vi "ROI info.vi"(6 "ROI info in":T7={"beads track"=[], "Public"={"标题名"="", "文件路径"=path "", "通道名"=[], "ROI Descriptor out"={"Global Rectangle"=[], "Contours"=[]}, "cali end"=0.0, "array piezo"=[], "LUT_R"=[], " ROI descriptors "=[{"Global Rectangle"=[0, 0, 0, 0], "Contours"=[{"ID"=enum."External", "Type"=12, "Coordinates"=[0, 0, 0, 0, 0]}]}, {"Global Rectangle"=[26, 104, 126, 204], "Contours"=[{"ID"=enum."External", "Type"=12, "Coordinates"=[26, 104, 126, 204, 0]}]}, {"Global Rectangle"=[99, 99, 201, 201], "Contours"=[{"ID"=enum."External", "Type"=12, "Coordinates"=[200, 200, 100, 100, 0]}]}], "tdms ref"=refnum, "分子长度(um)"=0.0, "ROI num"=0, "ROI size num"=[], "测量模式"=enum."force clamp"}, "beads info"=[]} {"Public"."ROI descriptors"."Contours"."Type" items=["No Selection", "Point", "Line", "Rectangle", "Oval", "Polygon", "Freehand Region", "Annulus", "Unused2", "Unused3", "Broken Line", "Freehand Line", "Rotated Rectangle"]; "Public"."ROI Descriptor out"."Contours"."Type" items=["No Selection", "Point", "Line", "Rectangle", "Oval", "Polygon", "Freehand Region", "Annulus", "Unused2", "Unused3", "Broken Line", "Freehand Line", "Rotated Rectangle"]; "beads track"."centroid"."Y Centroid" format="%.2f"; "beads track"."centroid"."X Centroid" format="%.2f"; "beads track"."ROI Des out"."Contours"."Type" items=["No Selection", "Point", "Line", "Rectangle", "Oval", "Polygon", "Freehand Region", "Annulus", "Unused2", "Unused3", "Broken Line", "Freehand Line", "Rotated Rectangle"]}, 7 "action":T8, 8 "error in (no error)":errorcluster caption="错误输入（无错误）", 9 "Public":T1={"标题名"="", "文件路径"=path "", "通道名"=[], "ROI Descriptor out"={"Global Rectangle"=[], "Contours"=[]}, "cali end"=0.0, "array piezo"=[], "LUT_R"=[], " ROI descriptors "=[{"Global Rectangle"=[0, 0, 0, 0], "Contours"=[{"ID"=enum."External", "Type"=12, "Coordinates"=[0, 0, 0, 0, 0]}]}, {"Global Rectangle"=[26, 104, 126, 204], "Contours"=[{"ID"=enum."External", "Type"=12, "Coordinates"=[26, 104, 126, 204, 0]}]}, {"Global Rectangle"=[99, 99, 201, 201], "Contours"=[{"ID"=enum."External", "Type"=12, "Coordinates"=[200, 200, 100, 100, 0]}]}], "tdms ref"=refnum, "分子长度(um)"=0.0, "ROI num"=0, "ROI size num"=[], "测量模式"=enum."force clamp"} {"ROI descriptors"."Contours"."Type" items=["No Selection", "Point", "Line", "Rectangle", "Oval", "Polygon", "Freehand Region", "Annulus", "Unused2", "Unused3", "Broken Line", "Freehand Line", "Rotated Rectangle"]; "ROI Descriptor out"."Contours"."Type" items=["No Selection", "Point", "Line", "Rectangle", "Oval", "Polygon", "Freehand Region", "Annulus", "Unused2", "Unused3", "Broken Line", "Freehand Line", "Rotated Rectangle"]}, 10 "beads track":T6[](array[typedef]) {"centroid"."Y Centroid" format="%.2f"; "centroid"."X Centroid" format="%.2f"; "ROI Des out"."Contours"."Type" items=["No Selection", "Point", "Line", "Rectangle", "Oval", "Polygon", "Freehand Region", "Annulus", "Unused2", "Unused3", "Broken Line", "Freehand Line", "Rotated Rectangle"]}, 11 "beads info":T4[](array[typedef])) -> (0 "error out":errorcluster caption="错误输出", 2 "ROI info out":T7={"beads track"=[], "Public"={"标题名"="", "文件路径"=path "", "通道名"=[], "ROI Descriptor out"={"Global Rectangle"=[], "Contours"=[]}, "cali end"=0.0, "array piezo"=[], "LUT_R"=[], " ROI descriptors "=[{"Global Rectangle"=[0, 0, 0, 0], "Contours"=[{"ID"=enum."External", "Type"=12, "Coordinates"=[0, 0, 0, 0, 0]}]}, {"Global Rectangle"=[26, 104, 126, 204], "Contours"=[{"ID"=enum."External", "Type"=12, "Coordinates"=[26, 104, 126, 204, 0]}]}, {"Global Rectangle"=[99, 99, 201, 201], "Contours"=[{"ID"=enum."External", "Type"=12, "Coordinates"=[200, 200, 100, 100, 0]}]}], "tdms ref"=refnum, "分子长度(um)"=0.0, "ROI num"=0, "ROI size num"=[], "测量模式"=enum."force clamp"}, "beads info"=[]} {"Public"."ROI descriptors"."Contours"."Type" items=["No Selection", "Point", "Line", "Rectangle", "Oval", "Polygon", "Freehand Region", "Annulus", "Unused2", "Unused3", "Broken Line", "Freehand Line", "Rotated Rectangle"]; "Public"."ROI Descriptor out"."Contours"."Type" items=["No Selection", "Point", "Line", "Rectangle", "Oval", "Polygon", "Freehand Region", "Annulus", "Unused2", "Unused3", "Broken Line", "Freehand Line", "Rotated Rectangle"]; "beads track"."centroid"."Y Centroid" format="%.2f"; "beads track"."centroid"."X Centroid" format="%.2f"; "beads track"."ROI Des out"."Contours"."Type" items=["No Selection", "Point", "Line", "Rectangle", "Oval", "Polygon", "Freehand Region", "Annulus", "Unused2", "Unused3", "Broken Line", "Freehand Line", "Rotated Rectangle"]})   [LabVIEW 2017]
doc: "本VI 是功能性全局变量，用来代替ROI info 四处乱跑的局域变量。\n暂时有初始化，读，写 3个功能。\nVI必须被设置为不可重入，以免出现执行中篡改的现象。"
uses:
  Bead info action.ctl
  vision test/ROI info.ctl
  Bead track.ctl
  beads public.ctl
  record mode.ctl
  bead info.ctl
  <vilib>/vision/Image Controls.llb/IMAQ Image.ctl
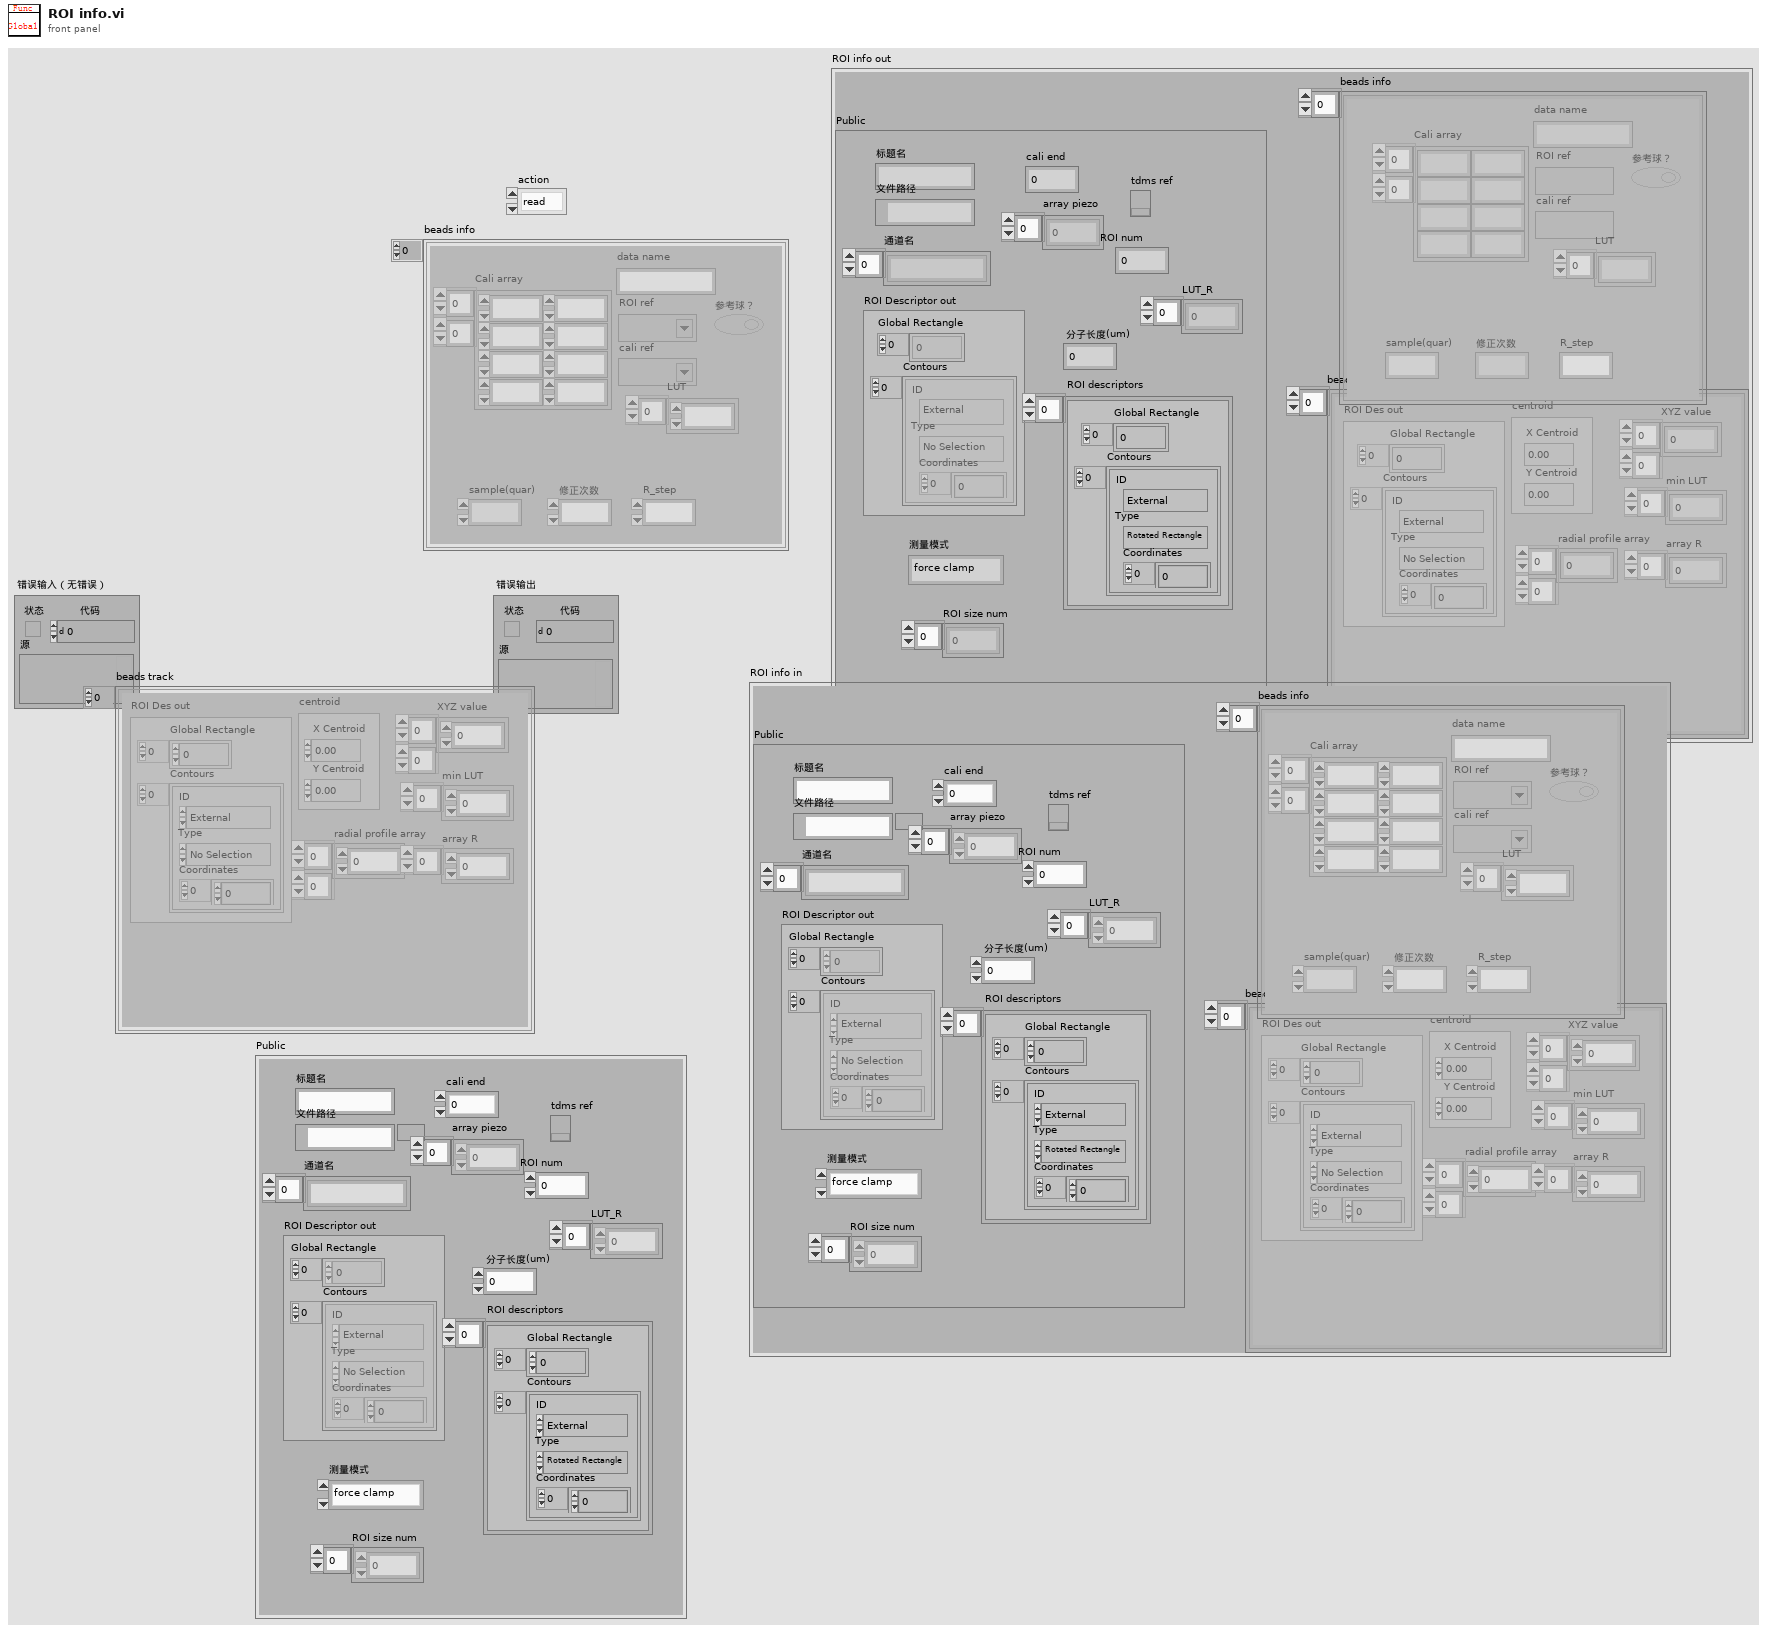
[diagram p1: front panel]
types:
  T1 = typedef "beads public.ctl" = cluster{"标题名":string, "文件路径":path, "通道名":string[], "ROI Descriptor out":T2, "cali end":dbl, "array piezo":dbl[], "LUT_R":dbl[], " ROI descriptors ":T2[], "tdms ref":refnum<k34>, "分子长度(um)":dbl, "ROI num":i32, "ROI size num":i32[], "测量模式":T3}
  T2 = typedef "ROI Descriptor" = cluster{"Global Rectangle":i32[], "Contours":cluster{"ID":enum32{"External", "Internal"}, "Type":u32, "Coordinates":i32[]}[]}
  T3 = typedef "record mode.ctl" = enum16{"force ramp", "force clamp", "user-defined", "force-mixed"}
  T4 = typedef "bead info.ctl" = cluster{"data name":string, "ROI ref":T5, "cali ref":T5, "参考球？":bool, "LUT":dbl[], "Cali array":dbl[][], "修正次数":i32, "R_step":dbl, "sample(quar)":i32}
  T5 = typedef "IMAQ Image.ctl" = refnum<image>
  T6 = typedef "Bead track.ctl" = cluster{"XYZ value":dbl[][], "radial profile array":dbl[][], "min LUT":dbl[], "ROI Des out":T2, "array R":dbl[], "centroid":cluster{"X Centroid":sgl, "Y Centroid":sgl}}
  T7 = typedef "ROI info.ctl" = cluster{"beads track":T6[], "Public":T1, "beads info":T4[]}
  T8 = typedef "Bead info action.ctl" = enum16{"read", "write track", "intial", "write info", "write all", "write public"}
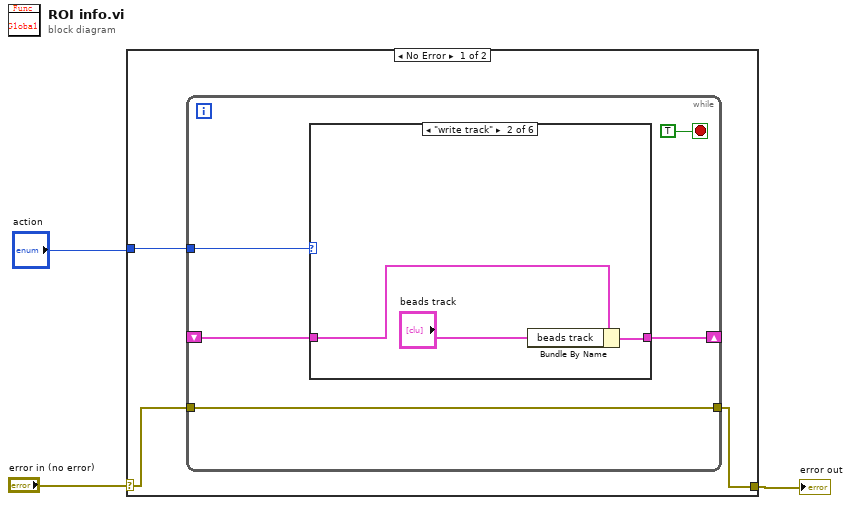
[diagram p0: block diagram]
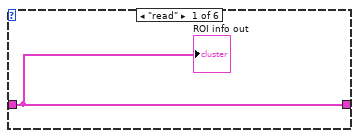
[diagram p2: hidden frame]
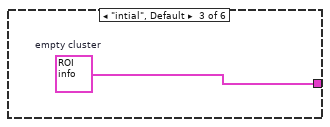
[diagram p3: hidden frame]
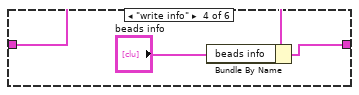
[diagram p4: hidden frame]
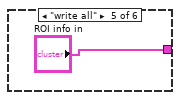
[diagram p5: hidden frame]
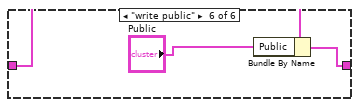
[diagram p6: hidden frame]
diagram:
  n1 = case shown="No Error" "error in (no error)" {
    selector: "error in (no error)" -> [w5 w24]
    tunnel: [w4 w24] -> w2
    tunnel: "action" -> [w6 _]
    frame No Error {
      n2 = while {
        tunnel: w6 -> [w11]
        shift-right: [w10] -> _
        shift-left: _ -> [w9]
        tunnel: w5 -> [w7]
        tunnel: [w7] -> w4
        stop <- TRUE stop-if-true
        n3 = case shown="\"write track\"" w11 {
          tunnel: [w12 w15 w16 w19 "ROI info in" w23] -> w10
          tunnel: w9 -> [w12 w13 _ w17 _ w21]
          frame "read" {
            "ROI info out" <- w12
          }
          frame "write track" {
            n4 = Bundle By Name(cluster=w13, "beads track"="beads track") -> (w15:T7)
          }
          frame "intial", Default {
            w16 = T7 {"beads track"=[], "Public"={"标题名"="", "文件路径"=path "", "通道名"=[], "ROI Descriptor out"={"Global Rectangle"=[], "Contours"=[]}, "cali end"=0.0, "array piezo"=[], "LUT_R"=[], " ROI descriptors "=[], "tdms ref"=refnum, "分子长度(um)"=0.0, "ROI num"=0, "ROI size num"=[], "测量模式"=enum."force ramp"}, "beads info"=[]}  # empty cluster
          }
          frame "write info" {
            n5 = Bundle By Name(cluster=w17, "beads info"="beads info") -> (w19:T7)
          }
          frame "write all" {
          }
          frame "write public" {
            n6 = Bundle By Name(cluster=w21, "Public"="Public") -> (w23:T7)
          }
        }
      }
    }
    frame Error {
    }
  }
  "error out" <- w2
